vi "Get Section Names.vi"(8 "error in (no error)":errorcluster, 11 "Config in":T1) -> (0 "error out":errorcluster, 1 "Section Names":string[](array[string]), 3 "Config out":T1)   [LabVIEW 2022 SP3, in "LabVIEW-Config.lvlib"]
uses:
  LabVIEW-Config.lvlib
  Config.ctl
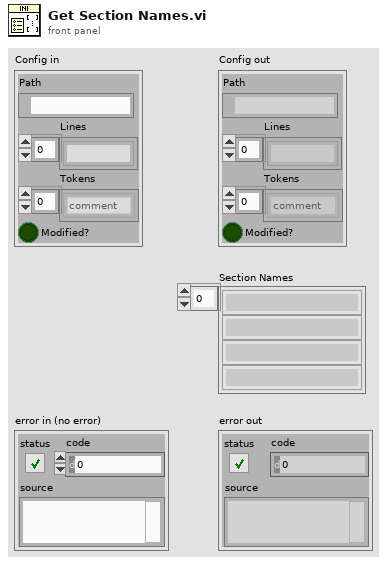
[diagram p1: front panel]
types:
  T1 = typedef "LabVIEW-Config.lvlib/Config.ctl" = cluster{"Path":path, "Lines":string[], "Tokens":enum8{"comment", "section", "key"}[], "Modified?":bool}
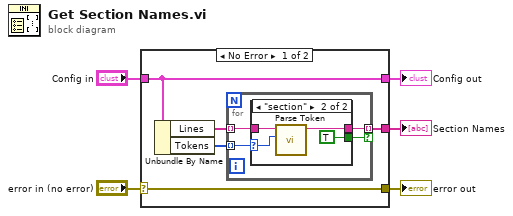
[diagram p0: block diagram]
diagram:
  n1 = case shown="No Error" "error in (no error)" {
    selector: "error in (no error)" -> [w7 w20]
    tunnel: "Config in" -> [w6 w19]
    tunnel: [w8 _] -> w4
    tunnel: [w7 w20] -> w3
    tunnel: [w6 w19] -> w1
    frame No Error {
      n2 = Unbundle By Name(w6) -> ("Lines"=w9:string[], "Tokens"=w10:enum8{"comment", "section", "key"}[])
      n3 = for {
        tunnel: w10 -> [w14] mode=indexing
        tunnel: w9 -> [w13] mode=indexing
        tunnel: [w12] -> w8 mode=indexing if=w11
        n4 = case shown="\"section\"" w14 {
          selector: w14 -> [_ w16]
          tunnel: w13 -> [_ w17]
          tunnel: [_ w15] -> w12
          tunnel: [_ TRUE] -> w11
          frame "comment", "key" {
          }
          frame "section" {
            n5 = call "Parse Token.vi"("Token"=w16, "Line"=w17) -> ("Name"=w15:string)  [unwired: 8 in, 1 out]
          }
        }
      }
    }
    frame Error {
    }
  }
  "error out" <- w3
  "Config out" <- w1
  "Section Names" <- w4
